vi "Process_New_Calls.vi"(8 "error in (no error)":errorcluster, 10 "Car Calls in":T1, 11 "Elevator Fleet in":T2) -> (0 "error out":errorcluster, 3 "Elevator Fleet out":T2)   [LabVIEW 2026]
uses:
  Controls/Door_Status_Enum.ctl
  Controls/Occupy_Status.ctl
  Controls/Floor_Status.ctl
  Controls/Motion_Status_Enum.ctl
  Controls/Car_Calls_Status.ctl
  Controls/Hall_Calls_Status.ctl
  Controls/Elevator_Status.ctl
  Controls/Elevator_Fleet.ctl
  Controls/Car_Calls.ctl
panel:
  out "Car Calls out":T1
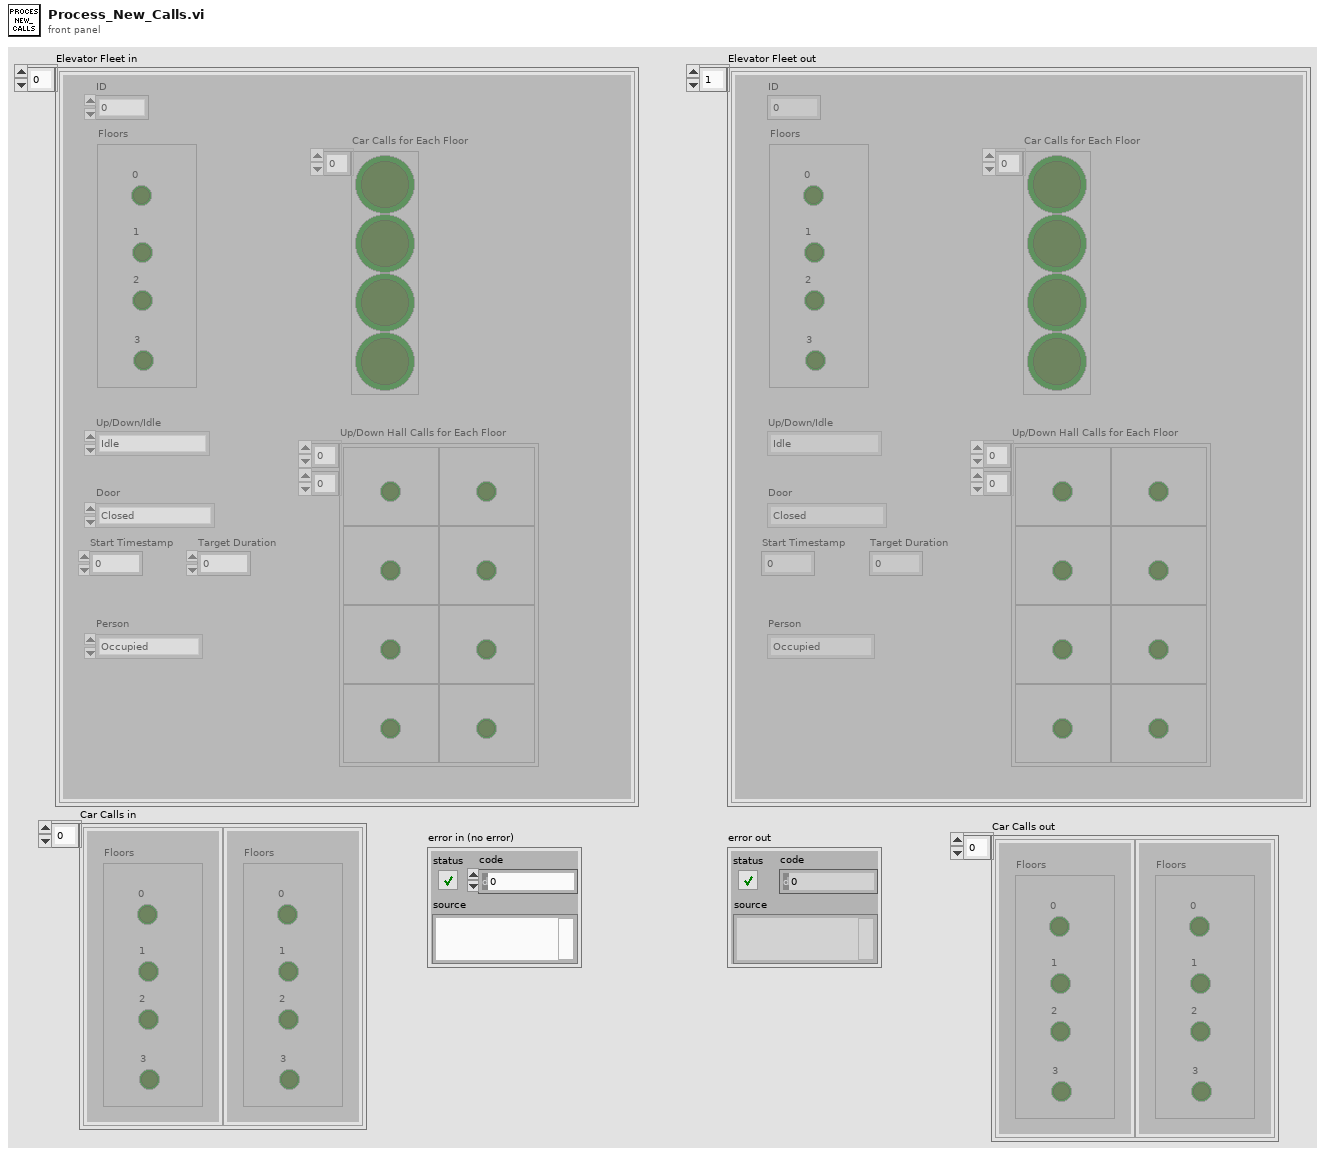
[diagram p1: front panel]
types:
  T1 = typedef "Car_Calls.ctl" = cluster{"Floors":cluster{"0":bool, "1":bool, "2":bool, "3":bool}}[]
  T2 = typedef "Elevator_Fleet.ctl" = T3[]
  T3 = typedef "Elevator_Status.ctl" = cluster{"Door":T4, "Person":T5, "Floors":T6, "Up/Down/Idle":T7, "Car Calls for Each Floor":T8, "Up/Down Hall Calls for Each Floor":T9, "ID":i32, "Start Timestamp":u32, "Target Duration":dbl}
  T4 = typedef "Door_Status_Enum.ctl" = enum16{"Closed", "Open", "Opening", "Closing"}
  T5 = typedef "Occupy_Status.ctl" = enum16{"Occupied", "Empty"}
  T6 = typedef "Floor_Status.ctl" = cluster{"0":bool, "1":bool, "2":bool, "3":bool}
  T7 = typedef "Motion_Status_Enum.ctl" = enum16{"Idle", "Up", "Down"}
  T8 = typedef "Car_Calls_Status.ctl" = bool[]
  T9 = typedef "Hall_Calls_Status.ctl" = cluster{bool}[][]
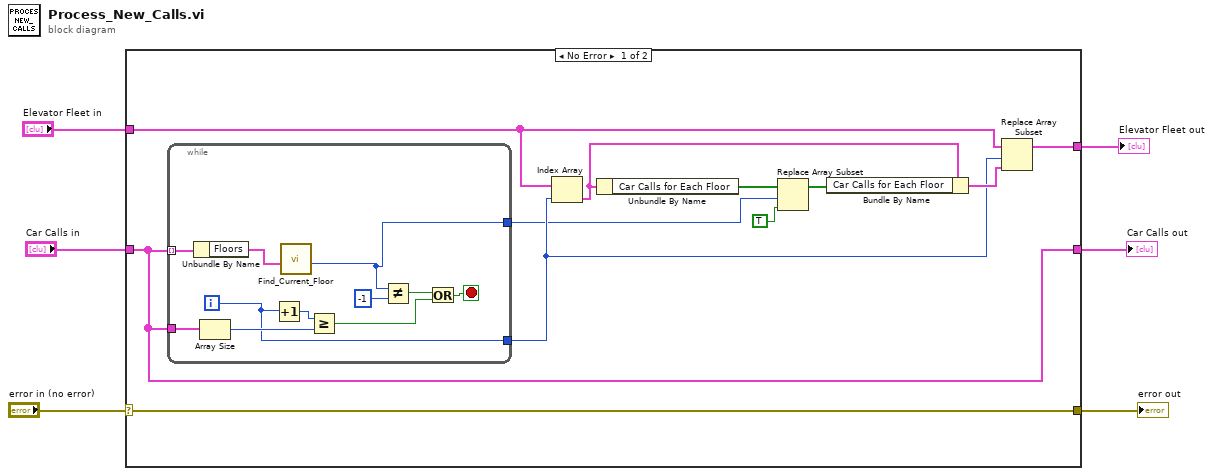
[diagram p0: block diagram]
diagram:
  n1 = case shown="No Error" "error in (no error)" {
    selector: "error in (no error)" -> [w10 w31]
    tunnel: [w17 w30] -> w6
    tunnel: "Elevator Fleet in" -> [w15 w30]
    tunnel: "Car Calls in" -> [w9 w29]
    tunnel: [w10 w31] -> w2
    tunnel: [w9 w29] -> w1
    frame No Error {
      n2 = while {
        tunnel: w9 -> [w22] mode=indexing
        tunnel: w9 -> [w25]
        tunnel: [w21] -> w8
        tunnel: [w18] -> w7
        i -> [w21]
        stop <- w26 stop-if-true
        n3 = Unbundle By Name(w22) -> ("Floors"=w19:cluster{"0":bool, "1":bool, "2":bool, "3":bool})
        n4 = Array Size(array=w25) -> (size(s)=w24:i32)
        n5 = Increment(x=w21) -> (x+1=w20:i32)
        n6 = call "Find_Current_Floor.vi"("Floors"=w19) -> ("Current Floor"=w18:i32)  [unwired: 7 in, 3 out]
        n7 = Greater Or Equal?(x=w20, y=w24) -> (x >= y?=w23:bool)
        n8 = Not Equal?(x=w18, y=-1) -> (x != y?=w27:bool)
        n9 = Or(x=w27, y=w23) -> (x .or. y?=w26:bool)
      }
      n10 = Index Array(array=w15, index=w8) -> (element=w14:T3)
      n11 = Unbundle By Name(w14) -> ("Car Calls for Each Floor"=w12:T8)
      n12 = Replace Array Subset(array=w12, new element=TRUE ("new element/subarray"), index=w7) -> (w11:T8)
      n13 = Bundle By Name(cluster=w14, "Car Calls for Each Floor"=w11) -> (w16:T3)
      n14 = Replace Array Subset(array=w15, new element=w16, index=w8) -> (w17:T2)
    }
    frame Error {
    }
  }
  "Elevator Fleet out" <- w6
  "error out" <- w2
  "Car Calls out" <- w1
